vi "Marker_Following_Vi.vi"() -> ()   [LabVIEW 2019]
uses:
  <vilib>/Platform/TimedLoop/XDataNode/timing_clust.ctl
  <vilib>/Platform/TimedLoop/XDataNode/nitl_modes.ctl
  <vilib>/Platform/TimedLoop/XDataNode/wakeup.ctl
  <vilib>/FPGAPlugInAG/sbRIO-9629/niLvFpga_Open_sbRIO-9629.vi
  <vilib>/rvi/interface/common/dynamic/niFpgaDynamicAddResources.vi
  <vilib>/imath/engines/lvmath2/RunTimeEngine/Managers/WorkSpace/UID Generator.vi
  <vilib>/imath/engines/lvmath2/RunTimeEngine/IndexRead/NIMS V(S).vi
  <instcachedir>/0/NIMS V(S)_0488751826AF41519A22953C041130DC.lvgen/NIMS V(S)_0488751826AF41519A22953C041130DC_000.vi
  <vilib>/imath/engines/lvmath2/RunTimeEngine/BuiltInFunctions/atan2/NIMS_atan2.vi
  <instcachedir>/0/NIMS_atan2_A91AA4A7D42247EDBE8F76DB99AF04A4.lvgen/NIMS_atan2_A91AA4A7D42247EDBE8F76DB99AF04A4_000.vi
  <vilib>/imath/engines/lvmath2/RunTimeEngine/RunTimeType/NIMS_RunTimeType_From StrictType (excl LVString).vi
  <instcachedir>/0/NIMS_RunTimeType_From StrictType (excl LVString)_D8AFBA86A94845AAA577C895450664BD.lvgen/NIMS_RunTimeType_From StrictType (excl LVString)_D8AFBA86A94845AAA577C895450664BD_000.vi
  <vilib>/imath/engines/lvmath2/RunTimeEngine/ErrorHandling/NIMS_Create Error From Enums.vi
  <vilib>/imath/engines/lvmath2/RunTimeEngine/LocalVariableDefStatement/MC_LocalVariableDefStatement_Display.vi
  <vilib>/imath/engines/lvmath2/RunTimeEngine/BuiltInFunctions/atan/NIMS_atan(C).vi
  <instcachedir>/0/NIMS_atan(C)_0A85D365582D4E8AB3874BC9125E138E.lvgen/NIMS_atan(C)_0A85D365582D4E8AB3874BC9125E138E_001.vi
  <vilib>/imath/engines/lvmath2/RunTimeEngine/BuiltInFunctions/cross/NIMS_cross(GV,GV).vi
  <instcachedir>/0/NIMS_cross(GV,GV)_6F1F1C643EFF41C8A983D972A94A5A15.lvgen/NIMS_cross(GV,GV)_6F1F1C643EFF41C8A983D972A94A5A15_000.vi
  <vilib>/imath/engines/lvmath2/RunTimeEngine/BuiltInFunctions/norm/NIMS_norm(GV,DBL).vi
  <instcachedir>/0/NIMS_norm(GV,DBL)_4A8B6F23BC0A47549B8AB805006257D9.lvgen/NIMS_norm(GV,DBL)_4A8B6F23BC0A47549B8AB805006257D9_000.vi
  <vilib>/imath/engines/lvmath2/RunTimeEngine/ArithmeticOperatorToken/NIMS_ArithmeticOperator_multmx-internal.vi
  <instcachedir>/0/NIMS_ArithmeticOperator_multmx-internal_9E91BA3A2DCB4083AAD724A04442A6F7.lvgen/NIMS_ArithmeticOperator_multmx-internal_9E91BA3A2DCB4083AAD724A04442A6F7_004.vi
  <vilib>/imath/engines/lvmath2/RunTimeEngine/BuiltInFunctions/cos/NIMS_cos(C).vi
  <instcachedir>/0/NIMS_cos(C)_BED070B05FDB4939A63CB05E18805866.lvgen/NIMS_cos(C)_BED070B05FDB4939A63CB05E18805866_001.vi
  <vilib>/imath/engines/lvmath2/RunTimeEngine/BuiltInFunctions/sin/NIMS_sin(C).vi
  <instcachedir>/0/NIMS_sin(C)_6504C6AC704B4661870B0E93397B11C4.lvgen/NIMS_sin(C)_6504C6AC704B4661870B0E93397B11C4_001.vi
  <vilib>/imathl/engines/lvmath/Functions/Error Handling/Create Error.vi
  <vilib>/imath/engines/lvmath2/RunTimeEngine/ArithmeticOperatorToken/NIMS_ArithmeticOperator_multmx(M,CV)-internal.vi
  <instcachedir>/0/NIMS_ArithmeticOperator_multmx(M,CV)-internal_2C55777844884EEDB828A940D397C7D0.lvgen/NIMS_ArithmeticOperator_multmx(M,CV)-internal_2C55777844884EEDB828A940D397C7D0_002.vi
  <instcachedir>/0/NIMS_norm(GV,DBL)_4A8B6F23BC0A47549B8AB805006257D9.lvgen/NIMS_norm(GV,DBL)_4A8B6F23BC0A47549B8AB805006257D9_001.vi
  <vilib>/imath/engines/lvmath2/RunTimeEngine/Managers/SymbolTable/Clear UID.vi
  <vilib>/imath/engines/lvmath2/RunTimeEngine/NodeEndStatement/NIMS_NodeEndStatement_Output.vi
  <instcachedir>/0/NIMS_NodeEndStatement_Output_53EC0D466D134D7ABD903AC30B43404B.lvgen/NIMS_NodeEndStatement_Output_53EC0D466D134D7ABD903AC30B43404B_001.vi
  <vilib>/imath/engines/lvmath2/RunTimeEngine/ErrorHandling/NIMS_Finalize Error.vi
  <vilib>/Utility/error.llb/Error Cluster From Error Code.vi
  <vilib>/rvi/errors/niLvFpgaAdjustHostInterfaceError.vi
  <vilib>/FPGAPlugInAG/Dynamic/niLvFpga_Close_Dynamic.vi
  <vilib>/rvi/interface/nirviOpenFPGA/nirviOpenFPGA.xnode
  FPGA Bitfiles/fcmsinglesection_FPGATarget_CloseLoopMotorTu_eGt+d+EV+VE.lvbitx
  Close_Loop_Motor_Tune.vi
  <vilib>/platform/TimedLoop/XDataNode/XDataNode.xnode
  <vilib>/rvi/interface/nirviReadWriteControl/nirviReadWriteControl.xnode
  <vilib>/rvi/interface/nirviCloseFPGA/nirviCloseFPGA.xnode
  NiFpgaLv.dll
  <vilib>/rvi/interface/Simulation/niFpgaSimulationCallBeginRW.vi
  <vilib>/imath/engines/lvmath2/RunTimeEngine/Managers/SymbolTable/NIMS_WorkSpace.lvlib
  <vilib>/Platform/TimedLoop/XDataNode/XDNodeRunTimeDep.lvlib
panel:
  out "error out 2":errorcluster
  out "L1 (m)":dbl
  out "L2 (m)":dbl
  out "L3 (m)":dbl
  out "Theta 1":dbl
  out "Theta 2":dbl
  out "Theta 3":dbl
  in  "Position Reset":bool
  out "output variable":dbl
  out "output variable 2":dbl
  out "output variable 3":dbl
  out "alpha":dbl
  out "L_v":dbl
  in  "Desired Tip position (m)":dbl[](array[numeric])
  out "data out 2":string
  out "FRAME 2":string
  out "LED ID 2":i32
  out "Y Position(mm) marker 48":dbl
  out "X Position(mm) marker 48":dbl
  out "Z Position(mm) marker 48":dbl
  out "Actual Tip Coordinates(m)":dbl[](array[numeric])
  out "Error":dbl[](array[numeric])
  out "L_v (error)":dbl
  out "alpha (error)":dbl
  out "Theta 1 (error)":dbl
  out "Theta 2 (error)":dbl
  out "Theta 3 (error)":dbl
  in  "Position Reset 2_e":bool
  in  "Motor1_KP":sgl
  in  "Motor2_KP":sgl
  in  "Motor3_KP":sgl
  out "Error Indicator":bool
  in  "Kp":dbl[](array[numeric])
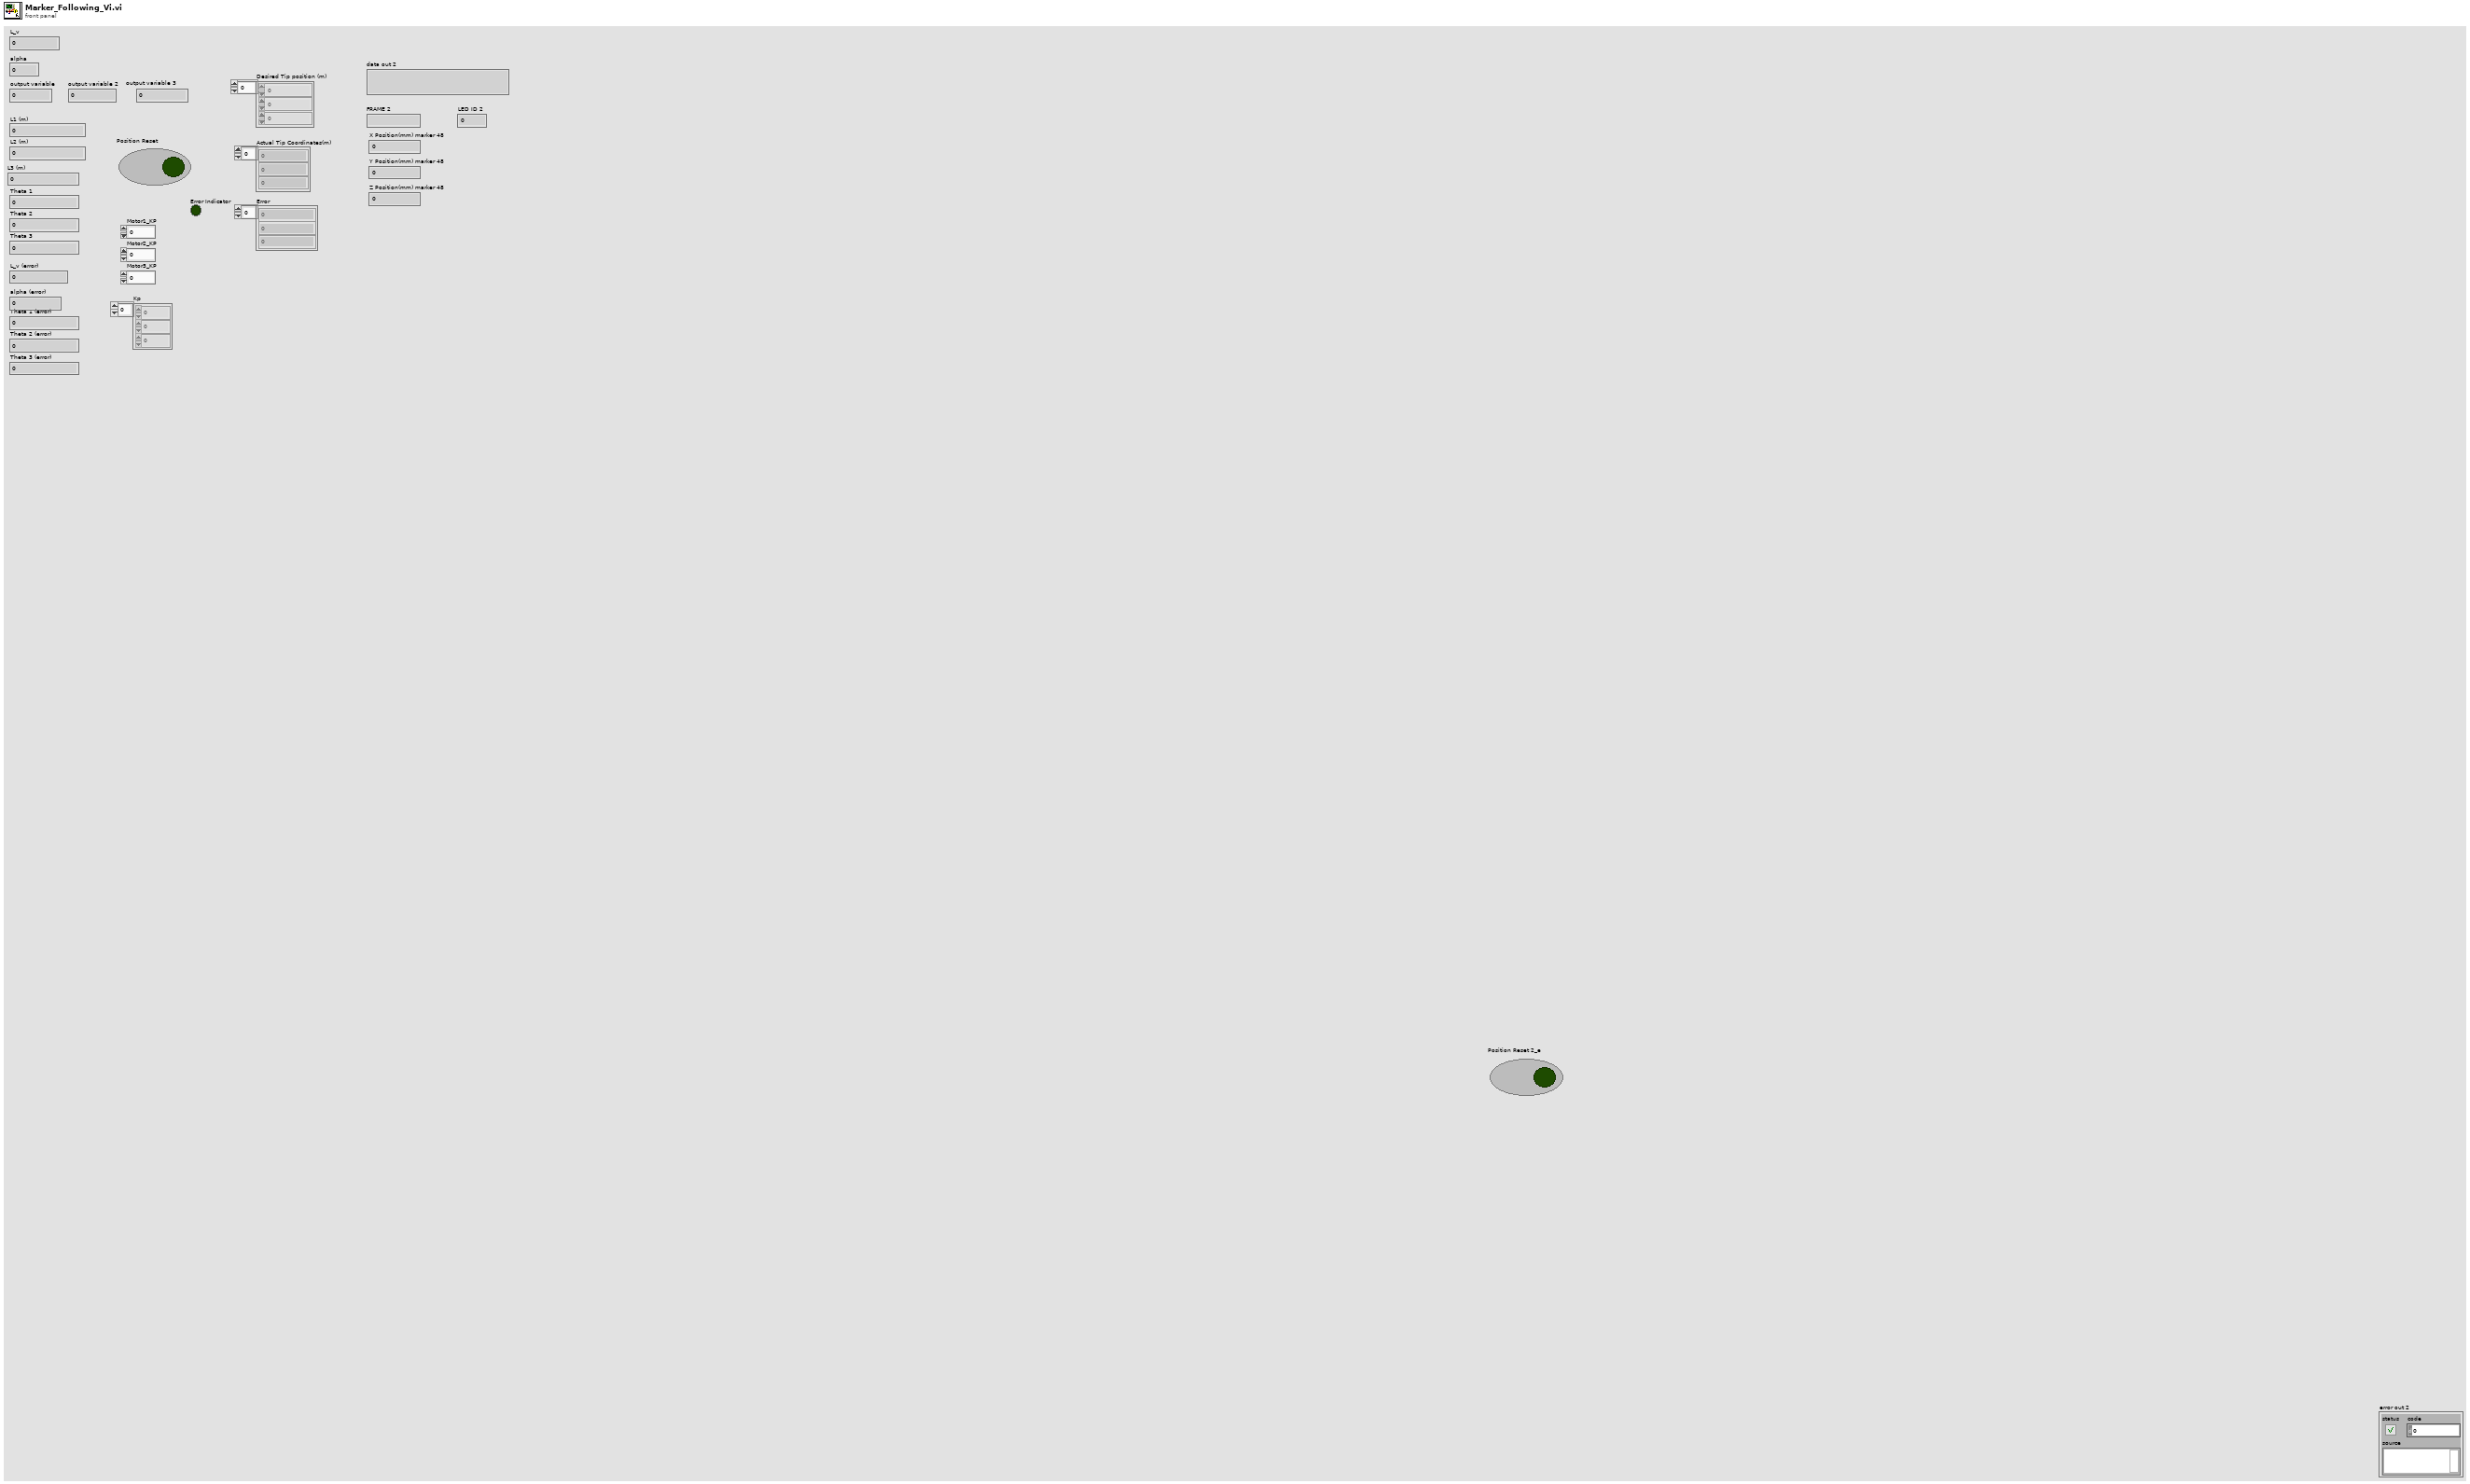
[diagram p1: front panel]
types:
  T1 = typedef "XDNodeRunTimeDep.lvlib/timing_clust.ctl" = cluster{"Expected End [f-1]":u64, "Actual End [f-1]":u64, "Finished Late? [f-1]":bool, "Expected End [i-1]":u64, "Actual End [i-1]":u64, "Finished Late? [i-1]":bool, "Expected Start [i]":u64, "Actual Start [i]":u64, "Expected Start [f]":u64, "Actual Start [f]":u64, "Source Name":string, "Structure Name":string, "Period":i64, "Deadline":i64, "Offset":i64, "Start":i64, "Priority":i32, "Timeout":i32, "Mode":T2, "Wakeup Reason":T3, "Error":errorcluster, "Source Type":string, "Secondary Source Type":string, "Global End Time":u64, "Global Start Time":u64, "Frame Duration":u64, "Iteration Duration":u64, "Assigned CPU":i32, "I/O Scan Engine Mode":u32}
  T2 = typedef "XDNodeRunTimeDep.lvlib/nitl_modes.ctl" = enum32{"No Change", "Process missed periods, maintain original phase", "Discard missed periods, maintain original phase", "Process missed periods, ignore original phase", "Discard missed periods, ignore original phase"}
  T3 = typedef "XDNodeRunTimeDep.lvlib/wakeup.ctl" = enum32{"Normal", "Aborted", "Asynchronous wakeup", "Timing source error", "Timed loop error", "Timeout"}
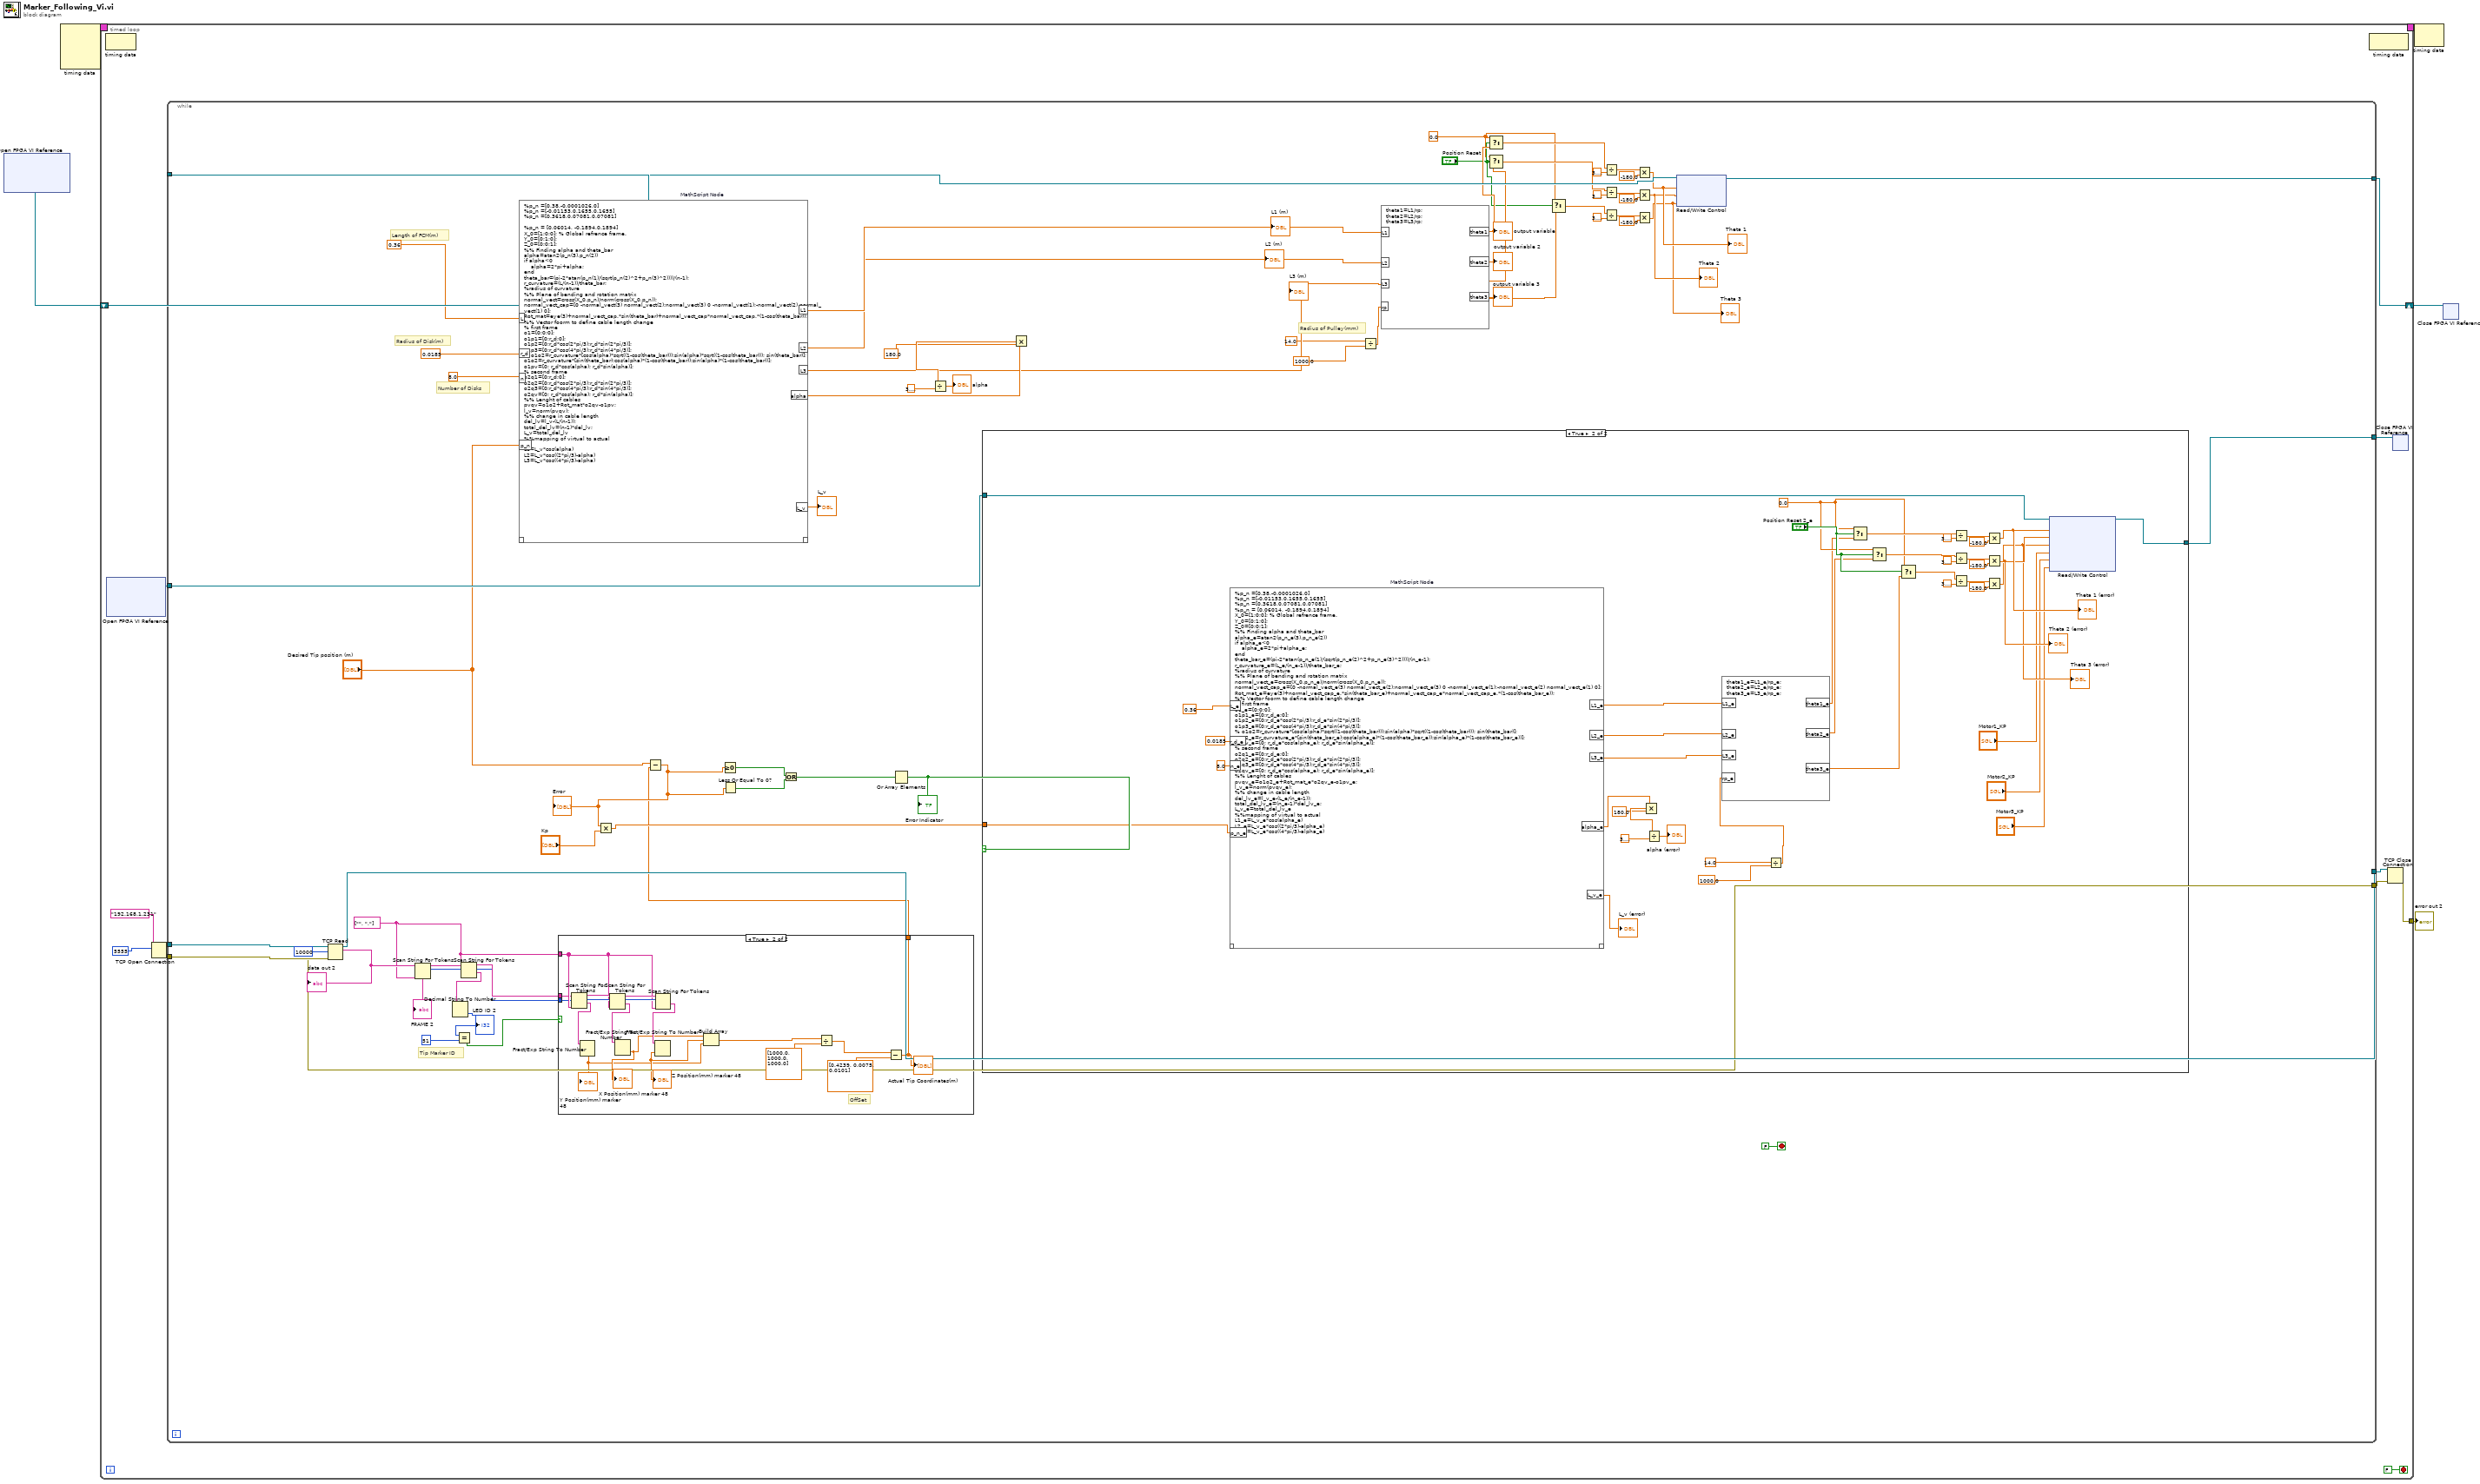
[diagram p0: block diagram]
diagram:
  n1 = xnode "Open FPGA VI Reference"() -> ("FPGA VI Reference Out"=w3:refnum<k20>)  [unwired: 2 in, 1 out]
  n2 = node-c288() -> (w2:T1)  [unwired: 4 in]
  n3 = timed-loop {
    timing: w2 -> [_]
    timing-out: [_] -> w1
    tunnel: [w12] -> w4
    shift-right: [w17] -> w5
    shift-left: w3 -> [w9]
    stop <- FALSE stop-if-true
    n4 = node-c288() -> ()  [unwired: 1 in, 1 out]
    n5 = xnode "Open FPGA VI Reference"() -> ("FPGA VI Reference Out"=w7:refnum<k20>)  [unwired: 2 in, 1 out]
    n6 = TCP Open Connection(address="192.168.1.231", remote port or service name=u16 5555) -> (connection ID=w13:refnum<k5>, error out=w14:errorcluster)  [unwired: 3 in]
    n7 = while {
      tunnel: w9 -> [w79]
      tunnel: [w78] -> w17
      tunnel: w14 -> [w42]
      tunnel: w13 -> [w41]
      tunnel: [w40] -> w11
      tunnel: [w39] -> w10
      tunnel: [w31] -> w8
      tunnel: w7 -> [w30]
      stop <- FALSE stop-if-true
      w22 = string[] ["", ","] ("delimiters (\\s,\\t,\\r,\\n)")
      w61 = 0.0 ("t")
      # "Tip Marker ID"
      # "Length of FCM(m)"
      # "Radius of Disk(m)"
      # "Number of Disks"
      # "Radius of Pulley(mm)"
      n8 = TCP Read(connection ID=w41, bytes to read=10000, error in (no error)=w42) -> (connection ID out=w40:refnum<k5>, data out=w24:string, error out=w39:errorcluster)  [unwired: 2 in]
      "data out 2" <- w24
      n9 = Scan String For Tokens(6:w22, 9:w24) -> (1:→"FRAME 2":string, 2:w23:i32, 3:w45:string)  [unwired: 4 in, 1 out]
      n10 = Scan String For Tokens(6:w22, 8:w23, 9:w45) -> (1:w18:string, 2:w20:i32, 3:w21:string)  [unwired: 3 in, 1 out]
      n11 = Decimal String To Number(string=w18) -> (number=w19:i32)  [unwired: 2 in, 1 out]
      "LED ID 2" <- w19
      n12 = Equal?(x=w19, y=51) -> (x = y?=w43:bool)
      n13 = mathscript code="%p_n =[0.38,-0.0001026,0] \n%p_n =[-0.01153,0.1655,0.1655] \n%p_n =[0.3618,0.07081,0.07081] \n\n%p_n = [0.06014, -0.1894,0.1894]\nX_0=[1;0;0]; % Global refrence frame.\nY_0=[0;1;0];\nZ_0=[0;0;1];\n%% Finding alpha and theta_bar\nalpha=atan2(p_n(3),p_n(2))\nif alpha<0\n    alpha=2*pi+alpha;\nend\ntheta_bar=(pi-2*atan(p_n(1)/(sqrt(p_n(2)^2+p_n(3)^2))))/(n-1);\nr_curvature=(L/(n-1))/theta_bar; \n%radius of curvature\n%% Plane of bending and rotation matrix\nnormal_vect=cross(X_0,p_n)/norm(cross(X_0,p_n));\nnormal_vect_cap=[0 -normal_vect(3) normal_vect(2);normal_vect(3) 0 -normal_vect(1);-normal_vect(2) normal_vect(1) 0];\nRot_mat=eye(3)+normal_vect_cap.*sin(theta_bar)+normal_vect_cap*normal_vect_cap.*(1-cos(theta_bar));\n%% Vector foorm to define cable length change\n% first frame\no1=[0;0;0];\no1p1=[0;r_d;0];\no1p2=[0;r_d*cos(2*pi/3);r_d*sin(2*pi/3)];\no1p3=[0;r_d*cos(4*pi/3);r_d*sin(4*pi/3)];\n% o1o2=r_curvature*[cos(alpha)*sqrt((1-cos(theta_bar)));sin(alpha)*sqrt((1-cos(theta_bar))); sin(theta_bar)];\no1o2=r_curvature*[sin(theta_bar);cos(alpha)*(1-cos(theta_bar));sin(alpha)*(1-cos(theta_bar))];\no1pv=[0; r_d*cos(alpha); r_d*sin(alpha)];\n% second frame\no2q1=[0;r_d;0];\no2q2=[0;r_d*cos(2*pi/3);r_d*sin(2*pi/3)];\no2q3=[0;r_d*cos(4*pi/3);r_d*sin(4*pi/3)];\no2qv=[0; r_d*cos(alpha); r_d*sin(alpha)];\n%% Lenght of cables\npvqv=o1o2+Rot_mat*o2qv-o1pv;\nl_v=norm(pvqv);\n%% change in cable length\ndel_lv=l_v-(L/(n-1));\ntotal_del_lv=(n-1)*del_lv;\nL_v=total_del_lv\n%%mapping of virtual to actual\n\nL1=L_v*cos(alpha)\nL2=L_v*cos((2*pi/3)-alpha)\nL3=L_v*cos((4*pi/3)-alpha)"("L"=0.36 ("Length of the FCM (mm)"), "r_d"=0.0185, "n"=8.0 ("Number of Disks"), "p_n"="Desired Tip position (m)") -> ("L_v"=→"L_v":dbl, "alpha"=w54:dbl, "L1"=w51:dbl, "L2"=w50:dbl, "L3"=w49:dbl)  [unwired: 1 in, 1 out]
      "L1 (m)" <- w51
      "L2 (m)" <- w50
      "L3 (m)" <- w49
      n14 = case shown="True" w43 {
        tunnel: w21 -> [_ w704]
        tunnel: w20 -> [_ w703]
        tunnel: w22 -> [_ w705]
        tunnel: [_ w698] -> w25
        frame False {
        }
        frame True {
          # "OffSet"
          n15 = Scan String For Tokens(6:w705, 8:w703, 9:w704) -> (1:w708:string, 2:w711:i32, 3:w713:string)  [unwired: 3 in, 1 out]
          n16 = Fract/Exp String To Number(string=w708) -> (number=w696:dbl)  [unwired: 3 in, 1 out]
          "Y Position(mm) marker 48" <- w696
          n17 = Scan String For Tokens(6:w705, 8:w711, 9:w713) -> (1:w709:string, 2:w710:i32, 3:w712:string)  [unwired: 3 in, 1 out]
          n18 = Fract/Exp String To Number(string=w709) -> (number=w706:dbl)  [unwired: 3 in, 1 out]
          "X Position(mm) marker 48" <- w706
          n19 = Scan String For Tokens(6:w705, 8:w710, 9:w712) -> (1:w707:string)  [unwired: 3 in, 3 out]
          n20 = Fract/Exp String To Number(string=w707) -> (number=w697:dbl)  [unwired: 3 in, 1 out]
          "Z Position(mm) marker 48" <- w697
          n21 = Build Array(w706, w697, w696) -> (w702:dbl[])
          n22 = Divide(x=w702, y=dbl[] [1000.0, 1000.0, 1000.0]) -> (x/y=w700:dbl[])
          n23 = Subtract(x=w700, y=dbl[] [0.4239, 0.0075, 0.0101]) -> (x-y=w698:dbl[])
          "Actual Tip Coordinates(m)" <- w698
        }
      }
      n24 = Subtract(x="Desired Tip position (m)", y=w25) -> (x-y=w28:dbl[])
      "Error" <- w28
      n25 = Multiply(x=w28, y="Kp") -> (x*y=w27:dbl[])
      n26 = Greater Or Equal To 0?(x=w28) -> (x >= 0?=w38:bool[])
      n27 = Less Or Equal To 0?(x=w28) -> (x <= 0?=w37:bool[])
      n28 = Or(x=w38, y=w37) -> (x .or. y?=w36:bool[])
      n29 = Or Array Elements(Boolean array=w36) -> (logical OR=w35:bool)
      "Error Indicator" <- w35
      n30 = case shown="True" w35 {
        tunnel: w27 -> [_ w124]
        tunnel: [w83 w91] -> w31
        tunnel: w30 -> [w83 w90]
        frame False {
        }
        frame True {
          w98 = 0.0 ("t")
          n31 = mathscript code="%p_n =[0.38,-0.0001026,0] \n%p_n =[-0.01153,0.1655,0.1655] \n%p_n =[0.3618,0.07081,0.07081] \n%p_n = [0.06014, -0.1894,0.1894]\nX_0=[1;0;0]; % Global refrence frame.\nY_0=[0;1;0];\nZ_0=[0;0;1];\n%% Finding alpha and theta_bar\nalpha_e=atan2(p_n_e(3),p_n_e(2))\nif alpha_e<0\n    alpha_e=2*pi+alpha_e;\nend\ntheta_bar_e=(pi-2*atan(p_n_e(1)/(sqrt(p_n_e(2)^2+p_n_e(3)^2))))/(n_e-1);\nr_curvature_e=(L_e/(n_e-1))/theta_bar_e; \n%radius of curvature\n%% Plane of bending and rotation matrix\nnormal_vect_e=cross(X_0,p_n_e)/norm(cross(X_0,p_n_e));\nnormal_vect_cap_e=[0 -normal_vect_e(3) normal_vect_e(2);normal_vect_e(3) 0 -normal_vect_e(1);-normal_vect_e(2) normal_vect_e(1) 0];\nRot_mat_e=eye(3)+normal_vect_cap_e.*sin(theta_bar_e)+normal_vect_cap_e*normal_vect_cap_e.*(1-cos(theta_bar_e));\n%% Vector foorm to define cable length change\n% first frame\no1_e=[0;0;0];\no1p1_e=[0;r_d_e;0];\no1p2_e=[0;r_d_e*cos(2*pi/3);r_d_e*sin(2*pi/3)];\no1p3_e=[0;r_d_e*cos(4*pi/3);r_d_e*sin(4*pi/3)];\n% o1o2=r_curvature*[cos(alpha)*sqrt((1-cos(theta_bar)));sin(alpha)*sqrt((1-cos(theta_bar))); sin(theta_bar)];\no1o2_e=r_curvature_e*[sin(theta_bar_e);cos(alpha_e)*(1-cos(theta_bar_e));sin(alpha_e)*(1-cos(theta_bar_e))];\no1pv_e=[0; r_d_e*cos(alpha_e); r_d_e*sin(alpha_e)];\n% second frame\no2q1_e=[0;r_d_e;0];\no2q2_e=[0;r_d_e*cos(2*pi/3);r_d_e*sin(2*pi/3)];\no2q3_e=[0;r_d_e*cos(4*pi/3);r_d_e*sin(4*pi/3)];\no2qv_e=[0; r_d_e*cos(alpha_e); r_d_e*sin(alpha_e)];\n%% Lenght of cables\npvqv_e=o1o2_e+Rot_mat_e*o2qv_e-o1pv_e;\nl_v_e=norm(pvqv_e);\n%% change in cable length\ndel_lv_e=l_v_e-(L_e/(n_e-1));\ntotal_del_lv_e=(n_e-1)*del_lv_e;\nL_v_e=total_del_lv_e\n%%mapping of virtual to actual\nL1_e=L_v_e*cos(alpha_e)\nL2_e=L_v_e*cos((2*pi/3)-alpha_e)\nL3_e=L_v_e*cos((4*pi/3)-alpha_e)"("L_e"=0.36 ("L"), "r_d_e"=0.0185 ("r_d"), "n_e"=8.0 ("n"), "p_n_e"=w124) -> ("L_v_e"=→"L_v (error)":dbl, "alpha_e"=w119:dbl, "L1_e"=w117:dbl, "L2_e"=w116:dbl, "L3_e"=w115:dbl)  [unwired: 1 in, 1 out]
          n32 = Multiply(x=w119, y=180.0) -> (x*y=w121:dbl)
          n33 = Divide(x=w121, y=3.141592653589793) -> (x/y=→"alpha (error)":dbl)
          n34 = Divide(x=14.0 ("Radius of pulley (mm)"), y=1000.0) -> (x/y=w113:dbl)
          n35 = formula code="theta1_e=L1_e/rp_e;\ntheta2_e=L2_e/rp_e;\ntheta3_e=L3_e/rp_e;"("L1_e"=w117, "L2_e"=w116, "L3_e"=w115, "rp_e"=w113) -> ("theta1_e"=w94:dbl, "theta2_e"=w93:dbl, "theta3_e"=w92:dbl)
          n36 = Select(t=w98, s="Position Reset 2_e", f=w94) -> (s? t:f=w102:dbl)
          n37 = Select(t=w98, s="Position Reset 2_e", f=w93) -> (s? t:f=w101:dbl)
          n38 = Select(t=w98, s="Position Reset 2_e", f=w92) -> (s? t:f=w100:dbl)
          n39 = Divide(x=w102, y=3.141592653589793) -> (x/y=w110:dbl)
          n40 = Divide(x=w101, y=3.141592653589793) -> (x/y=w107:dbl)
          n41 = Divide(x=w100, y=3.141592653589793) -> (x/y=w104:dbl)
          n42 = Multiply(x=w110, y=-180.0) -> (x*y=w97:dbl)
          "Theta 1 (error)" <- w97
          n43 = Multiply(x=w107, y=-180.0) -> (x*y=w96:dbl)
          "Theta 2 (error)" <- w96
          n44 = Multiply(x=w104, y=-180.0) -> (x*y=w95:dbl)
          "Theta 3 (error)" <- w95
          n45 = xnode "Read/Write Control"("FPGA VI Reference In"=w90, "desired angle (error)"=w97, "desired angle 2(error)"=w96, "desired angle 3(error)"=w95, "Motor1_KP"="Motor1_KP", "Motor2_KP"="Motor2_KP", "Motor3_KP"="Motor3_KP") -> ("FPGA VI Reference Out"=w91:refnum<k20>)  [unwired: 1 in, 1 out]
        }
      }
      n46 = Multiply(x=w54, y=180.0) -> (x*y=w56:dbl)
      n47 = Divide(x=w56, y=3.141592653589793) -> (x/y=→"alpha":dbl)
      n48 = Divide(x=14.0, y=1000.0) -> (x/y=w81:dbl)
      n49 = formula code="theta1=L1/rp;\ntheta2=L2/rp;\ntheta3=L3/rp;"("L1"=w51, "L2"=w50, "L3"=w49, "rp"=w81) -> ("theta1"=w68:dbl, "theta2"=w65:dbl, "theta3"=w63:dbl)
      "output variable" <- w68
      "output variable 2" <- w65
      "output variable 3" <- w63
      n50 = Select(t=w61, s="Position Reset", f=w68) -> (s? t:f=w67:dbl)
      n51 = Select(t=w61, s="Position Reset", f=w65) -> (s? t:f=w66:dbl)
      n52 = Select(t=w61, s="Position Reset", f=w63) -> (s? t:f=w64:dbl)
      n53 = Divide(x=w67, y=3.141592653589793) -> (x/y=w76:dbl)
      n54 = Divide(x=w66, y=3.141592653589793) -> (x/y=w73:dbl)
      n55 = Divide(x=w64, y=3.141592653589793) -> (x/y=w70:dbl)
      n56 = Multiply(x=w76, y=-180.0) -> (x*y=w60:dbl)
      "Theta 1" <- w60
      n57 = Multiply(x=w73, y=-180.0) -> (x*y=w59:dbl)
      "Theta 2" <- w59
      n58 = Multiply(x=w70, y=-180.0) -> (x*y=w58:dbl)
      "Theta 3" <- w58
      n59 = xnode "Read/Write Control"("FPGA VI Reference In"=w79, "desired angle"=w60, "desired angle 2"=w59, "desired angle 3"=w58) -> ("FPGA VI Reference Out"=w78:refnum<k20>)  [unwired: 1 in, 1 out]
    }
    n60 = node-c288() -> ()  [unwired: 1 in, 1 out]
    n61 = TCP Close Connection(connection ID=w11, error in (no error)=w10) -> (error out=w12:errorcluster)  [unwired: 1 in, 1 out]
    n62 = xnode "Close FPGA VI Reference"("FPGA VI Reference In"=w8) -> ()  [unwired: 1 in, 1 out]
  }
  "error out 2" <- w4
  n63 = node-c288(w1) -> ()  [unwired: 1 out]
  n64 = xnode "Close FPGA VI Reference"("FPGA VI Reference In"=w5) -> ()  [unwired: 1 in, 1 out]
